vi "IRISS V2 Get Joint Out.vi"(5 "Left or Right Arm":i32(ring)=1 items=["Left Arm", "Right Arm"]) -> (0 "grasp":dbl, 1 "Joint Out Posit":dbl[](array[numeric]))   [LabVIEW 2016]
uses:
  EyeRobotDLL.dll
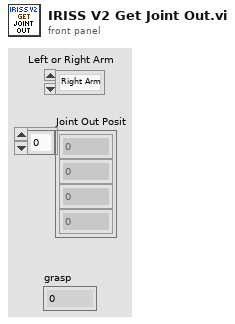
[diagram p1: front panel]
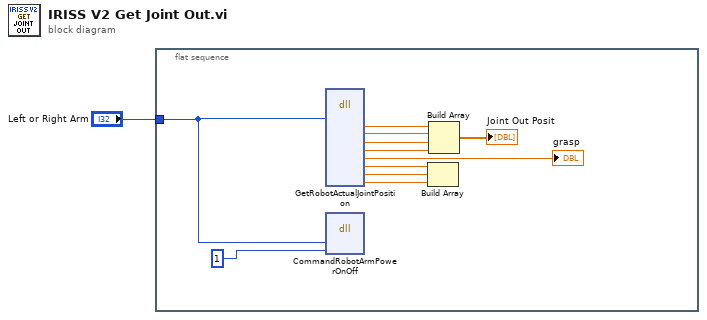
[diagram p0: block diagram]
diagram:
  n1 = flat-sequence {
    tunnel: "Left or Right Arm" -> [w10]
    frame #0 {
      n2 = dll-call lib="D:/IRISSoft LV2016 beta/Host Demo/Functions/EyeRobotDLL.dll" fn="GetRobotActualJointPosition"("armID"=w10) -> ("j0"=w9:dbl, "j1"=w8:dbl, "j2"=w7:dbl, "j3"=w6:dbl, "j4"=→"grasp":dbl, "j5"=w4:dbl, "j6"=w3:dbl, "j7"=w2:dbl)  [unwired: 13 in, 2 out]
      n3 = dll-call lib="D:/IRISSoft LV2016 beta/Host Demo/Functions/EyeRobotDLL.dll" fn="CommandRobotArmPowerOnOff"("id"=w10, "OnOff"=1) -> ()  [unwired: 6 in, 2 out]
      n4 = Build Array(w4, w3, w2) -> ()  [unwired: 1 out]
      n5 = Build Array(w9, w8, w7, w6) -> (→"Joint Out Posit":dbl[])
    }
  }
